vi "mWmotor_get_motor_para.vi"(8 "error in (no error)":errorcluster, 11 "VISA resource name":refnum<visa-resource-name>) -> (0 "error out":errorcluster, 2 "Current mortor parameters":cluster{"Velocity":dbl, "Acceleration":dbl}, 3 "VISA resource name out":refnum<visa-resource-name>)   [LabVIEW 2019]
panel:
  in  "milliseconds to wait":u32=100
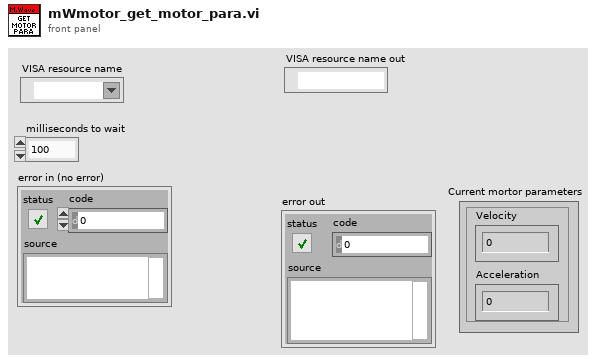
[diagram p1: front panel]
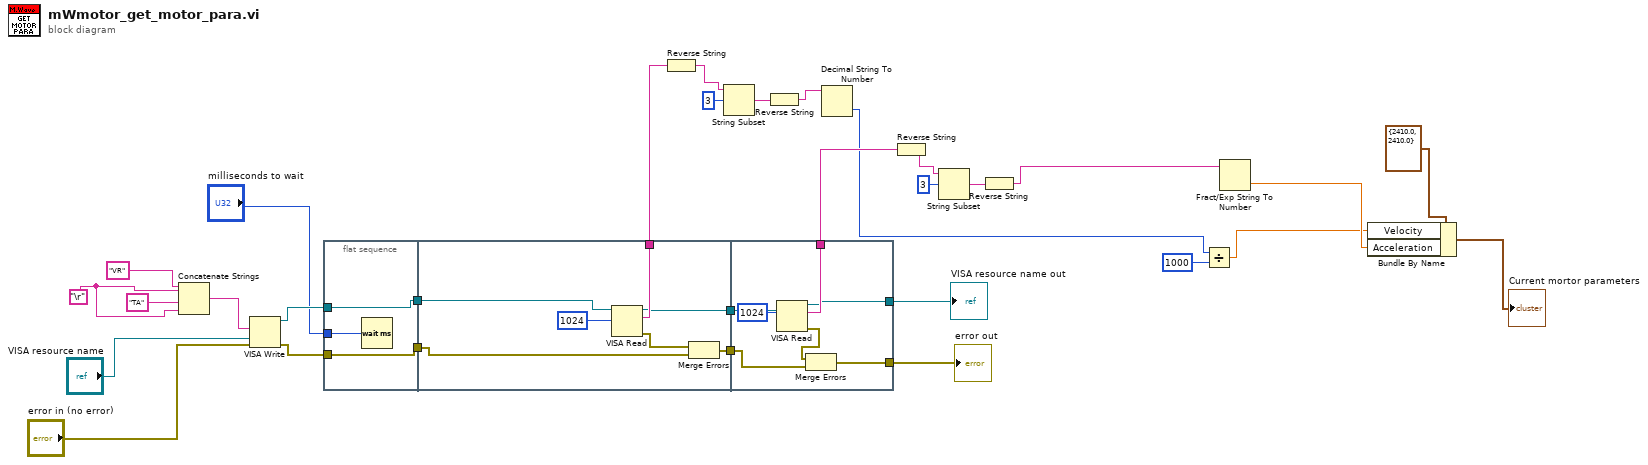
[diagram p0: block diagram]
diagram:
  w19 = "\r"
  n1 = Concatenate Strings("VR" ("string"), w19, "TA" ("string"), w19) -> (w31:string)
  n2 = VISA Write(VISA resource name="VISA resource name", write buffer=w31, error in (no error)="error in (no error)") -> (VISA resource name out=w27:refnum<visa-resource-name>, error out=w28:errorcluster)  [unwired: 1 out]
  n3 = flat-sequence {
    tunnel: w28 -> [w34]
    tunnel: w27 -> [w33]
    tunnel: "milliseconds to wait" -> [w32]
    tunnel: [w34] -> w14
    tunnel: [w33] -> w13
    tunnel: w14 -> [w36]
    tunnel: w13 -> [w40]
    tunnel: [w39] -> w12
    tunnel: [w38] -> w11
    tunnel: [w35] -> w10
    tunnel: w11 -> [w46]
    tunnel: w10 -> [w48]
    tunnel: [w47] -> w9
    tunnel: [w44] -> w8
    tunnel: [w43] -> w7
    frame #0 {
      n4 = Wait (ms)(milliseconds to wait=w32) -> ()  [unwired: 1 out]
    }
    frame #1 {
      n5 = VISA Read(VISA resource name=w40, byte count=u32 1024) -> (VISA resource name out=w38:refnum<visa-resource-name>, read buffer=w39:string, error out=w37:errorcluster)  [unwired: 1 in, 1 out]
      n6 = Merge Errors(w37, w36) -> (w35:errorcluster)
    }
    frame #2 {
      n7 = VISA Read(VISA resource name=w46, byte count=u32 1024) -> (VISA resource name out=w43:refnum<visa-resource-name>, read buffer=w44:string, error out=w45:errorcluster)  [unwired: 1 in, 1 out]
      n8 = Merge Errors(w45, w48) -> (w47:errorcluster)
    }
  }
  n9 = Reverse String(1:w12) -> (0:w23:string)
  n10 = String Subset(string=w23, offset (0)=3) -> (substring=w22:string)  [unwired: 1 in]
  n11 = Reverse String(1:w22) -> (0:w21:string)
  n12 = Decimal String To Number(string=w21) -> (number=w3:i32)  [unwired: 2 in, 1 out]
  n13 = Reverse String(1:w8) -> (0:w17:string)
  n14 = String Subset(string=w17, offset (0)=3) -> (substring=w18:string)  [unwired: 1 in]
  n15 = Reverse String(1:w18) -> (0:w6:string)
  n16 = Divide(x=w3, y=1000) -> (x/y=w1:dbl)
  n17 = Fract/Exp String To Number(string=w6) -> (number=w5:dbl)  [unwired: 3 in, 1 out]
  n18 = Bundle By Name(cluster=cluster{"Velocity":dbl, "Acceleration":dbl} {"Velocity"=2410.0, "Acceleration"=2410.0} ("Cluster"), "Velocity"=w1, "Acceleration"=w5) -> (→"Current mortor parameters":cluster{"Velocity":dbl, "Acceleration":dbl})
  "error out" <- w9
  "VISA resource name out" <- w7
